vi "acquireValue.vi"(8 "error in (no error)":errorcluster, 10 "nextSample?":bool, 11 "settingsAppliedDomeTcp in":refnum<class "settingsAppliedDomeTcp.lvclass">) -> (0 "error out":errorcluster, 1 "function return":i32, 2 "variantData":variant, 3 "settingsAppliedDomeTcp out":refnum<class "settingsAppliedDomeTcp.lvclass">)   [LabVIEW 2016, in "SALLV_AtDome_Messaging.lvlib" / "settingsAppliedDomeTcp.lvclass"]
uses:
  settingsAppliedDomeTcp.lvclass
  ts_sallv_AtDome/SALLV_AtDome.lvlib
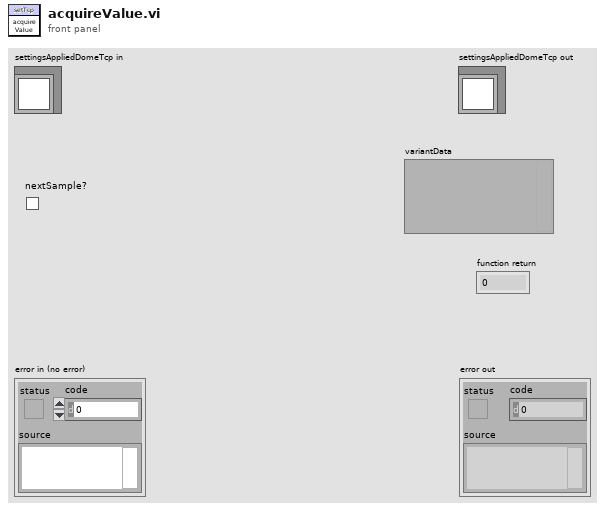
[diagram p1: front panel]
types:
  T1 = typedef "SALLV_AtDome.lvlib/logevent_settingsAppliedDomeTcp.ctl" = cluster{"ip":string, "portRange":i32, "readTimeout":sgl, "writeTimeout":sgl, "connectionTimeout":sgl, "priority":i32}
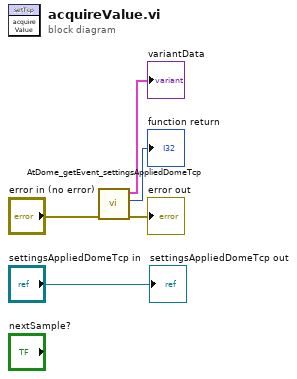
[diagram p0: block diagram]
diagram:
  n1 = call "AtDome_getEvent_settingsAppliedDomeTcp.vi"("error in (no error)"="error in (no error)") -> ("error out"=→"error out":errorcluster, "function return"=→"function return":i32, "logevent_settingsAppliedDomeTcp_Ctl out"=→"variantData":T1)  [unwired: 8 in]
  "settingsAppliedDomeTcp out" <- "settingsAppliedDomeTcp in"
